vi "STM Read Message (TCP).vi"(6 "Options":T2={"Ignore Timeout Error"=TRUE, "timeout ms (1000)"=1000}, 8 "error in":errorcluster, 11 "Connection Info":T4) -> (0 "error out":errorcluster, 1 "Name":T3, 2 "data string":string, 3 "Connection Info Out":T4, 4 "Data Info":T1, 5 "Timed Out?":bool)   [LabVIEW 2010]
doc: "This VI reads an incoming package of data from a host. This VI parses the package and extracts the data name and type as described in the meta data.\n\nFor the package to be parsed correctly, the meta data must be consistent in both the sender and the receiver. The data is packaged based on the existing meta data on the sender. \n\nUse the \"STM Read Meta Data\" and \"STM Write Meta Data\" VIs to ensure that both client and server have the same meta data.\n\nThe data is returned as a string. It is the responsibility of the user to cast it to the appropriate type."
uses:
  stm_TCP Connection Info.ctl
  stm_MetaDataElement.ctl
  stm_TCP Read Options.ctl
  stm_TCP Data Info.ctl
  NI STM.lvlib
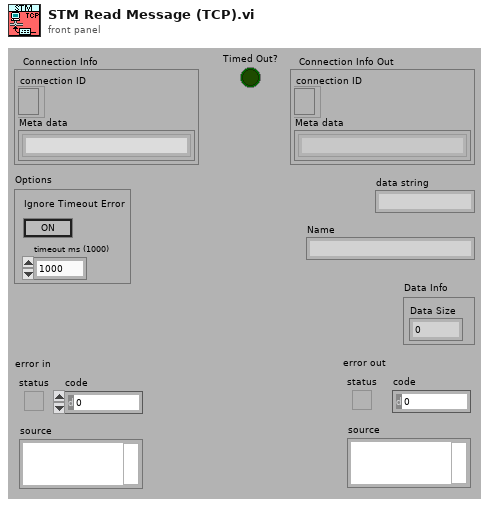
[diagram p1: front panel]
types:
  T1 = typedef "stm_TCP Data Info.ctl" = cluster{"Data Size":i32}
  T2 = typedef "stm_TCP Read Options.ctl" = cluster{"Ignore Timeout Error":bool, "timeout ms (1000)":i32}
  T3 = typedef "stm_MetaDataElement.ctl" = string
  T4 = typedef "stm_TCP Connection Info.ctl" = cluster{"connection ID":refnum<k5>, "Meta data":T3[]}
  T5 = typedef "NI STM.lvlib/MetaDataElement.ctl" = string
  T6 = typedef "NI STM.lvlib/TCP Connection Info.ctl" = cluster{"connection ID":refnum<k5>, "Meta data":T5[]}
  T7 = typedef "NI STM.lvlib/TCP Data Info.ctl" = cluster{"Data Size":i32}
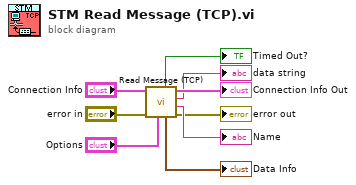
[diagram p0: block diagram]
diagram:
  n1 = call "Read Message (TCP).vi"("Options"="Options", "error in"="error in", "Connection Info"="Connection Info") -> ("error out"=→"error out":errorcluster, "Name"=→"Name":T5, "data string"=→"data string":string, "Connection Info Out"=→"Connection Info Out":T6, "Data Info"=→"Data Info":T7, "Timed Out?"=→"Timed Out?":bool)  [unwired: 3 in]
